vi "XY Galvo With Homography.vi"(0 "Exposure (ms)":dbl=10.0 format="%0.2p", 1 "Underscan /ms":dbl, 2 "Camera Delay /ms":dbl, 4 "Samples /Millisecond":dbl=10.0 format="%0.2p", 5 "Relax (ms)":dbl=10.0 format="%0.2p", 18 "Piezo Position (um)":dbl) -> (14 "Y Mirror Signal":dbl[](graph), 15 "Piezo Signal":dbl[](graph), 16 "Camera Signal":dbl[](graph), 17 "Laser Signal":dbl[](graph), 19 "Z Mirror Signal":dbl[](graph))   [LabVIEW 2016]
uses:
  controls/GlobalVariables.vi
  <vilib>/Analysis/NI_AALBase.lvlib
panel:
  out "Time Taken (ms)":dbl
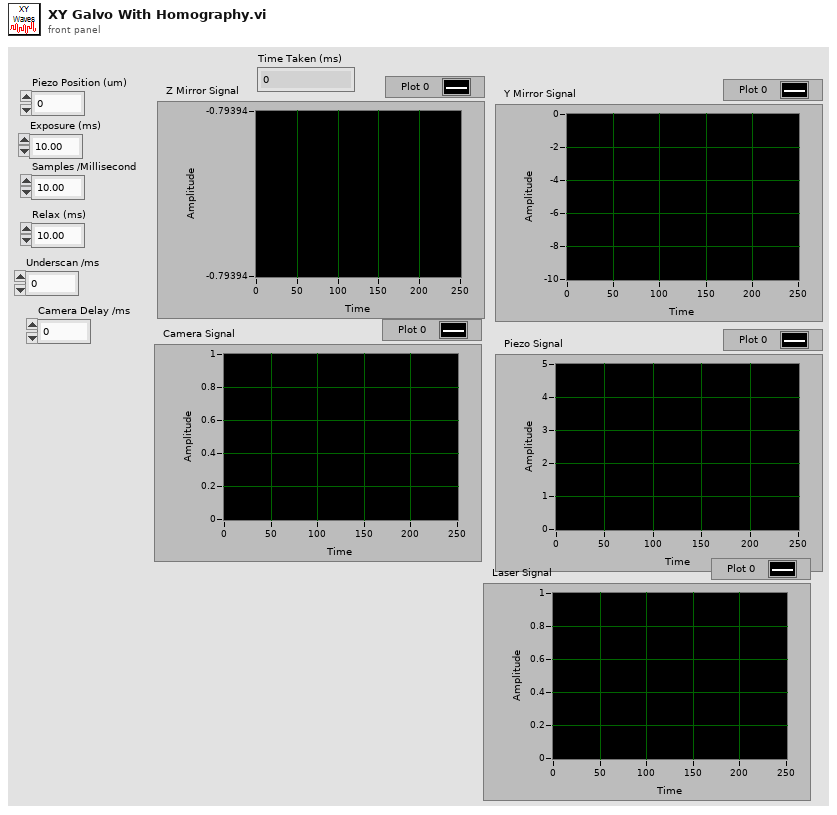
[diagram p1: front panel]
types:
  T1 = cluster{"Top Left":dbl[], "Top Right":dbl[], "Bottom Left":dbl[], "Bottom Right":dbl[]}
  T2 = typedef "NI_Matrix.lvlib/RealMatrix.ctl" = dbl[][]
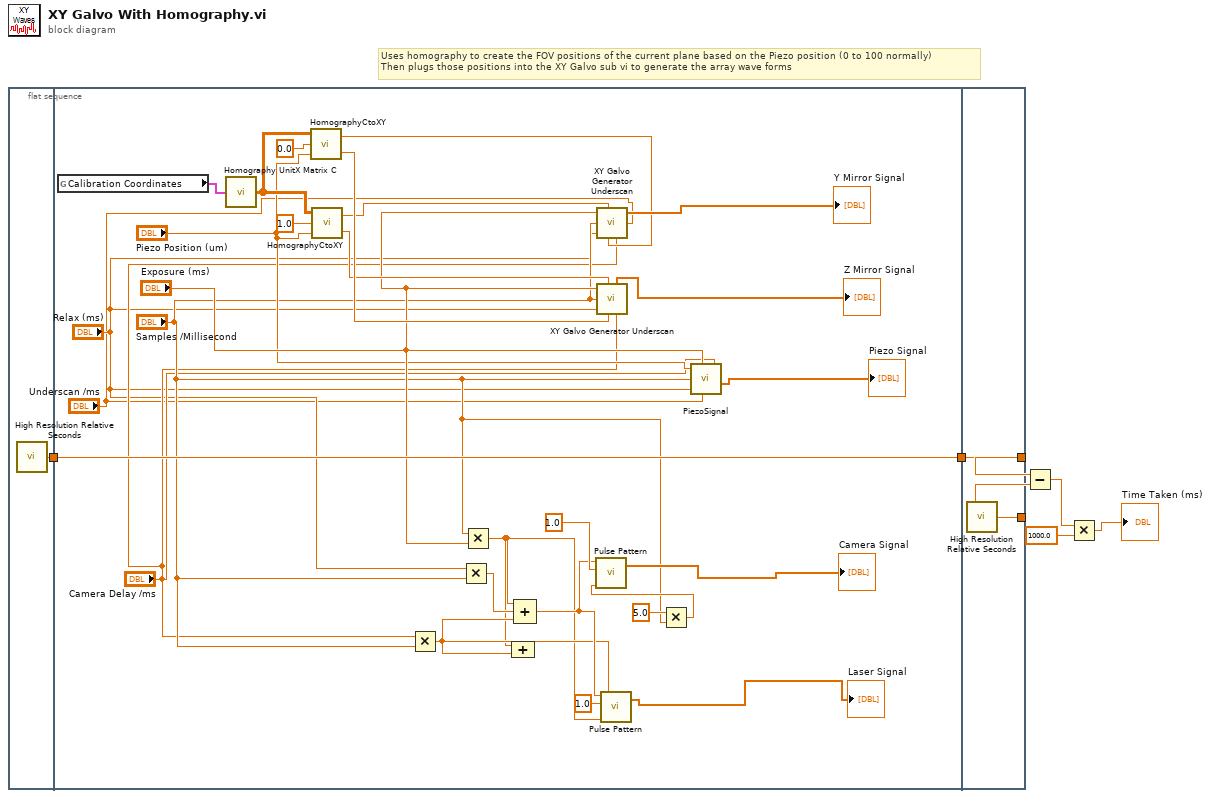
[diagram p0: block diagram]
diagram:
  # "Uses homography to create the FOV positions of the current plane based on the Piezo position (0 to 100 normally)\nThen plugs those positions into the XY Galvo sub vi to generate the array wave forms"
  n1 = flat-sequence {
    tunnel: [w8] -> w6
    tunnel: [w27] -> w7
    tunnel: w6 -> [w27]
    tunnel: w7 -> [w38]
    tunnel: [w38] -> w5
    tunnel: [w37] -> w4
    frame #0 {
      n2 = call <vilib>:"High Resolution Relative Seconds.vi"() -> ("relative seconds"=w8:dbl)
    }
    frame #1 {
      n3 = global read "GlobalVariables.vi" "Calibration Coordinates"() -> (w35:T1)
      n4 = call "Homography UnitX Matrix C.vi"("input cluster"=w35) -> ("C"=w32:T2)
      n5 = call "HomographyCtoXY.vi"("Y"="Piezo Position (um)", "X"=0.0, "C"=w32) -> ("Y"=w31:dbl, "X"=w29:dbl)
      n6 = call "HomographyCtoXY.vi"("Y"="Piezo Position (um)", "X"=1.0, "C"=w32) -> ("Y"=w30:dbl, "X"=w28:dbl)
      n7 = Multiply(x="Camera Delay /ms", y="Samples /Millisecond") -> (x*y=w21:dbl)
      n8 = Multiply(x="Relax (ms)", y="Samples /Millisecond") -> (x*y=w24:dbl)
      n9 = Multiply(x="Samples /Millisecond", y="Exposure (ms)") -> (x*y=w20:dbl)
      n10 = Compound Arithmetic op=ADD(w20, w21) -> ()  [unwired: 1 out]
      n11 = Compound Arithmetic op=ADD(w20, w24, w21) -> (w22:dbl)
      n12 = call "XY Galvo Generator Underscan.vi"("Exposure /ms"="Exposure (ms)", "FOV max / V"=w28, "Samples per ms"="Samples /Millisecond", "Relax /ms"="Relax (ms)", "FOV min/ V"=w29, "Underscan /ms"="Underscan /ms", "Delay /ms"="Camera Delay /ms") -> ("Signal"=→"Y Mirror Signal":dbl[])  [unwired: 2 in]
      n13 = call "XY Galvo Generator Underscan.vi"("Exposure /ms"="Exposure (ms)", "FOV max / V"=w30, "Samples per ms"="Samples /Millisecond", "Relax /ms"="Relax (ms)", "FOV min/ V"=w31, "Delay /ms"="Camera Delay /ms") -> ("Signal"=→"Z Mirror Signal":dbl[])  [unwired: 3 in]
      n14 = call <vilib>:"Pulse Pattern.vi"("width"=w20, "delay"=w21, "amplitude"=1.0, "samples"=w22) -> ("Pulse Pattern"=→"Laser Signal":dbl[])  [unwired: 1 out]
      n15 = Multiply(x=5.0, y="Samples /Millisecond") -> (x*y=w16:dbl)
      n16 = call <vilib>:"Pulse Pattern.vi"("width"=w16, "amplitude"=1.0, "samples"=w22) -> ("Pulse Pattern"=→"Camera Signal":dbl[])  [unwired: 1 in, 1 out]
      n17 = call "PiezoSignal.vi"("Piezo Position (um)"="Piezo Position (um)", "Exposure (ms)"="Exposure (ms)", "Samples /Millisecond"="Samples /Millisecond", "Relax (ms)"="Relax (ms)", "Underscan /ms"="Underscan /ms", "Camera Delay /ms"="Camera Delay /ms") -> ("Signal"=→"Piezo Signal":dbl[])  [unwired: 2 in]
    }
    frame #2 {
      n18 = call <vilib>:"High Resolution Relative Seconds.vi"() -> ("relative seconds"=w37:dbl)
    }
  }
  n19 = Subtract(x=w5, y=w4) -> (x-y=w3:dbl)
  n20 = Multiply(x=w3, y=1000.0) -> (x*y=→"Time Taken (ms)":dbl)
